vi "PolByteInfo.vi"(6 "error in (no error)":errorcluster, 9 "VISA resource name":refnum<visa-resource-name>="COM3") -> (0 "error out":errorcluster, 2 "Polhemus Info":T1, 3 "VISA resource name out":refnum<visa-resource-name>)   [LabVIEW 2009]
doc: "Gets general information about the current state of the Polhemus Fastrak including:\nUnits of output\nFormat of output\nStations plugged in and on\nByte order and list for each station output\n\nReturns all in cluster, 'Polhemus Info'"
uses:
  <vilib>/Instr/_visa.llb/VISA Configure Serial Port (Instr).vi
panel:
  out "Output Item List":string[](array[string])
  out "Active Station State":string
  out "Status":string
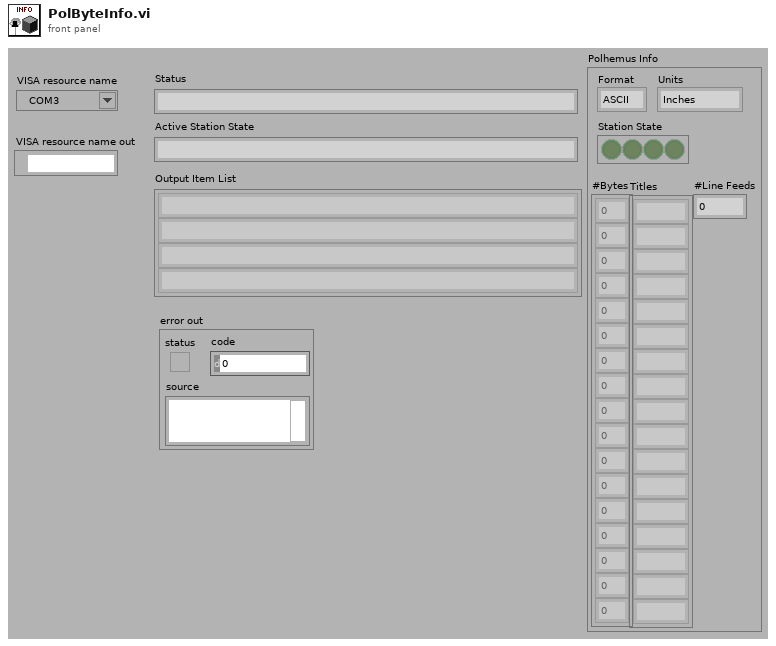
[diagram p1: front panel]
types:
  T1 = cluster{"#Bytes":i32[], "Titles":string[], "Format":enum16{"ASCII", "Binary"}, "Units":enum16{"Inches", "Centimeters"}, "Station State":bool[], "#Line Feeds":i32}
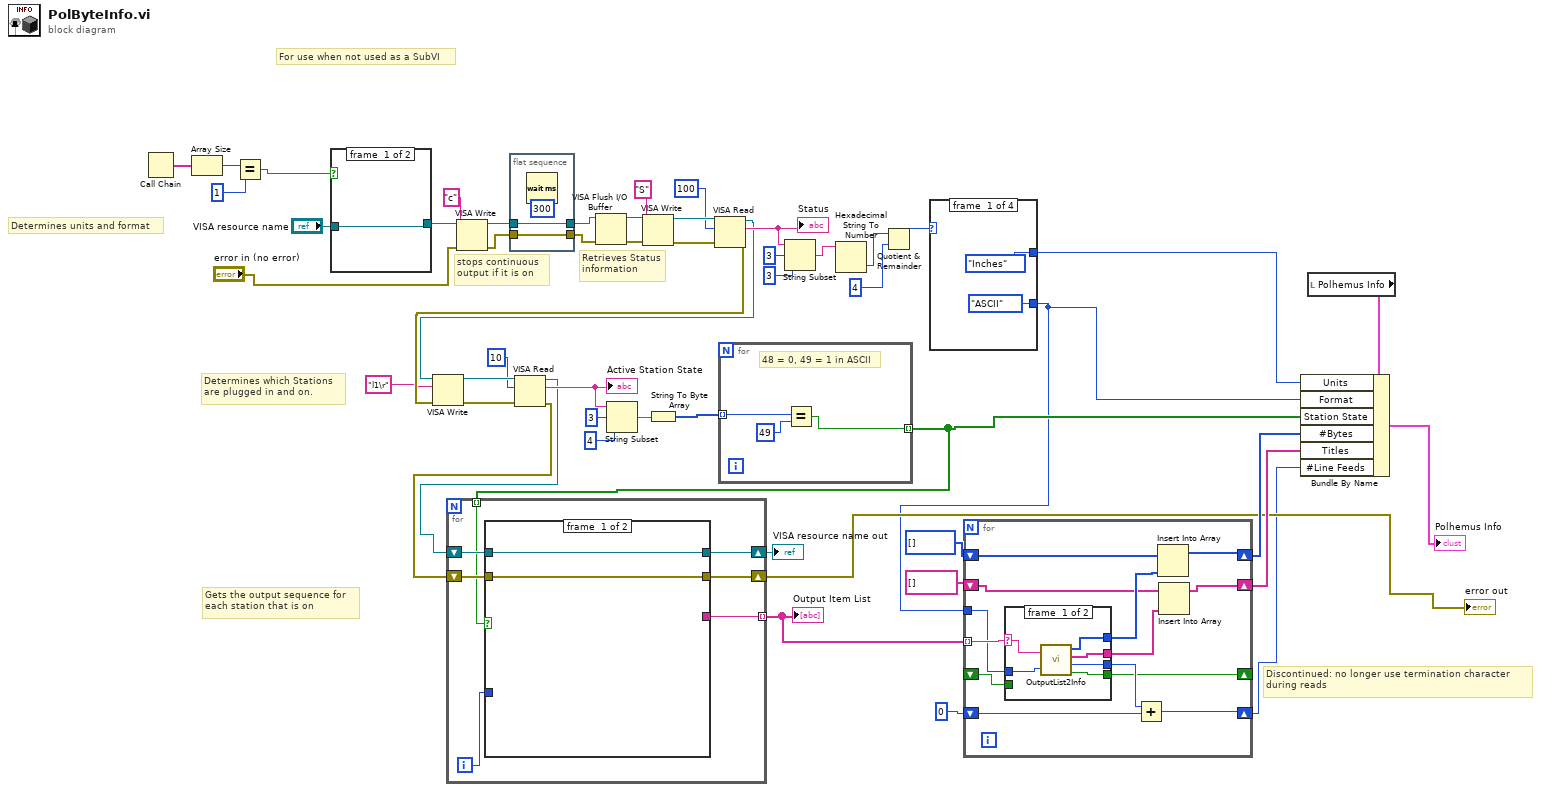
[diagram p0: block diagram]
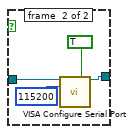
[diagram p2: hidden frame]
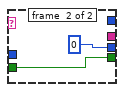
[diagram p3: hidden frame]
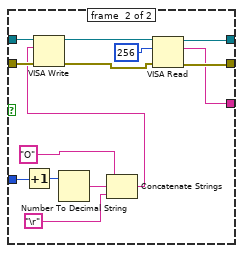
[diagram p4: hidden frame]
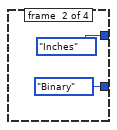
[diagram p5: hidden frame]
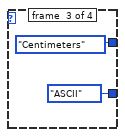
[diagram p6: hidden frame]
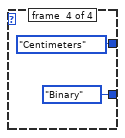
[diagram p7: hidden frame]
diagram:
  # "Discontinued: no longer use termination character\nduring reads"
  # "Gets the output sequence for\neach station that is on"
  # "For use when not used as a SubVI"
  # "Determines which Stations\nare plugged in and on."
  # "Determines units and format"
  # "Retrieves Status\ninformation"
  # "stops continuous\noutput if it is on"
  n1 = Call Chain() -> (call chain=w4:string[])
  n2 = Array Size(array=w4) -> (size(s)=w3:i32)
  n3 = Equal?(x=w3, y=1) -> (x = y?=w1:bool)
  n4 = case shown="False" w1 {
    tunnel: [w53 w57] -> w27
    tunnel: "VISA resource name" -> [w53 w56]
    frame #0 {
    }
    frame #1 {
      n5 = call-poly "VISA Configure Serial Port"("VISA resource name"=w56, "Enable Termination\nChar (T)"=TRUE ("Enable Termination\nChar (T)"), "baud rate (9600)"=u32 115200) -> ("VISA resource name out"=w57:refnum<visa-resource-name>)  [unwired: 11 in, 1 out]
    }
  }
  n6 = VISA Write(VISA resource name=w27, write buffer="c", error in (no error)="error in (no error)") -> (VISA resource name out=w8:refnum<visa-resource-name>, error out=w6:errorcluster)  [unwired: 1 out]
  n7 = flat-sequence {
    tunnel: w8 -> [w60]
    tunnel: [w60] -> w7
    tunnel: w6 -> [w59]
    tunnel: [w59] -> w5
    frame #0 {
      n8 = Wait (ms)(milliseconds to wait=u32 300) -> ()  [unwired: 1 out]
    }
  }
  n9 = VISA Flush I/O Buffer(VISA resource name=w7, error in (no error)=w5) -> (VISA resource name out=w50:refnum<visa-resource-name>, error out=w51:errorcluster)  [unwired: 1 in]
  n10 = VISA Write(VISA resource name=w50, write buffer="S", error in (no error)=w51) -> (VISA resource name out=w47:refnum<visa-resource-name>, error out=w48:errorcluster)  [unwired: 1 out]
  n11 = VISA Read(VISA resource name=w47, byte count=u32 100, error in (no error)=w48) -> (VISA resource name out=w37:refnum<visa-resource-name>, read buffer=w45:string, error out=w38:errorcluster)  [unwired: 1 out]
  "Status" <- w45
  n12 = VISA Write(VISA resource name=w37, write buffer="l1\r", error in (no error)=w38) -> (VISA resource name out=w35:refnum<visa-resource-name>, error out=w33:errorcluster)  [unwired: 1 out]
  n13 = VISA Read(VISA resource name=w35, byte count=u32 10, error in (no error)=w33) -> (VISA resource name out=w25:refnum<visa-resource-name>, read buffer=w32:string, error out=w24:errorcluster)  [unwired: 1 out]
  "Active Station State" <- w32
  n14 = String Subset(string=w32, offset (0)=3, length (rest)=4 ("length (rest)")) -> (substring=w29:string)
  n15 = String To Byte Array(string=w29) -> (unsigned byte array=w28:u8[])
  n16 = for {
    tunnel: w28 -> [w63] mode=indexing
    tunnel: [w61] -> w12 mode=indexing
    # "48 = 0, 49 = 1 in ASCII"
    n17 = Equal?(x=w63, y=u8 49) -> (x = y?=w61:bool)
  }
  n18 = for {
    tunnel: w12 -> [w68] mode=indexing
    shift-right: [w67] -> w23
    shift-left: w25 -> [w70]
    shift-right: [w66] -> w15
    shift-left: w24 -> [w69]
    tunnel: [w64] -> w16 mode=indexing
    i -> [w65]
    n19 = case shown="True" w68 {
      tunnel: w70 -> [w72 w86]
      tunnel: w69 -> [w71 w85]
      tunnel: [w72 w75] -> w67
      tunnel: [w71 w74] -> w66
      tunnel: w65 -> [_ w83]
      tunnel: [_ w73] -> w64
      frame #0 {
      }
      frame #1 {
        n20 = Increment(x=w83) -> (x+1=w82:i32)
        n21 = Number To Decimal String(number=w82) -> (decimal integer string=w81:string)  [unwired: 1 in]
        n22 = Concatenate Strings("O" ("string"), w81, "\r") -> (w79:string)
        n23 = VISA Write(VISA resource name=w86, write buffer=w79, error in (no error)=w85) -> (VISA resource name out=w78:refnum<visa-resource-name>, error out=w76:errorcluster)  [unwired: 1 out]
        n24 = VISA Read(VISA resource name=w78, byte count=u32 256, error in (no error)=w76) -> (VISA resource name out=w75:refnum<visa-resource-name>, read buffer=w73:string, error out=w74:errorcluster)  [unwired: 1 out]
      }
    }
  }
  "Output Item List" <- w16
  "VISA resource name out" <- w23
  "error out" <- w15
  n25 = String Subset(string=w45, offset (0)=3, length (rest)=3 ("length (rest)")) -> (substring=w42:string)
  n26 = Hexadecimal String To Number(string=w42) -> (number=w41:u32)  [unwired: 2 in, 1 out]
  n27 = Quotient & Remainder(x=w41, y=u32 4) -> (x-y*floor(x/y)=w39:u32)  [unwired: 1 out]
  n28 = case shown="3" w39 {
    tunnel: [enum16{"ASCII", "Binary"}."ASCII" ("Format") enum16{"ASCII", "Binary"}."Binary" ("Format") enum16{"ASCII", "Binary"}."ASCII" ("Format") enum16{"ASCII", "Binary"}."Binary" ("Format")] -> w11
    tunnel: [enum16{"Inches", "Centimeters"}."Inches" ("Units") enum16{"Inches", "Centimeters"}."Inches" ("Units") enum16{"Inches", "Centimeters"}."Centimeters" ("Units") enum16{"Inches", "Centimeters"}."Centimeters" ("Units")] -> w10
    frame #0 {
    }
    frame #1 {
    }
    frame #2 {
    }
    frame #3 {
    }
  }
  n29 = for {
    tunnel: w16 -> [w107] mode=indexing
    tunnel: w11 -> [w106]
    shift-right: [w97] -> w9
    shift-left: 0 ("#Reads In") -> [w98]
    shift-right: [w105] -> w17
    shift-left: i32[] [] ("Output Bytes") -> [w100]
    shift-right: [w103] -> w20
    shift-left: string[] [] ("Output Titles") -> [w101]
    shift-right: [w95] -> _
    shift-left: _ -> [w96]
    n30 = case shown="Default" w107 {
      selector: w107 -> [w110 _]
      tunnel: w106 -> [w113 _]
      tunnel: [w112 _] -> w102
      tunnel: [w111 _] -> w104
      tunnel: [w109 0 ("#Reads Out")] -> w99
      tunnel: [w108 w114] -> w95
      tunnel: w96 -> [_ w114]
      frame #0 {
        n31 = call "OutputList2Info.vi"("Output List String"=w110, "Format"=w113) -> ("Output Bytes"=w111:i32[], "Output Titles"=w112:string[], "#Reads Out"=w109:i32, "Ends with Terminator?"=w108:bool)
      }
      frame #1 {
      }
    }
    n32 = Add(x=w99, y=w98) -> (x+y=w97:i32)
    n33 = Insert Into Array(array=w100, new element=w104) -> (w105:i32[])  [unwired: 1 in]
    n34 = Insert Into Array(array=w101, new element=w102) -> (w103:string[])  [unwired: 1 in]
  }
  n35 = local read "Polhemus Info"() -> (w13:T1)
  n36 = Bundle By Name(cluster=w13, "Units"=w10, "Format"=w11, "Station State"=w12, "#Bytes"=w17, "Titles"=w20, "#Line Feeds"=w9) -> (→"Polhemus Info":T1)
